vi "Untitled4.vi"() -> ()   [LabVIEW 2020]
uses:
  HAL/Source/Config from JSON/Config from JSON.lvclass
  HAL/HAL-Devices/source/Configure Strategies/PCAN-USB Strategies/PCAN-USB Read-Write Raw CAN Frame Strategy/PCAN Read-Write Raw CAN Frame Strategy.lvclass
  HAL/Source/Communicator/Communicator.lvclass
  CANopen Response/CANopen Response Message.lvclass
  CANopen Master/CANopen Master.lvclass
  CANopen Message/CANopen Message.lvclass
  <vilib>/ProgressBar/Progress Bar Dialog.lvclass
  EDS-File-Viewer/source/Electronic Datasheet/Electronic Datasheet.lvclass
panel:
  out "Success":bool[](array[boolean])
  out "Objects List":string[](array[string])
  out "Values":variant[](array[variant])
  in  "Actual Values Button":bool
  out "Uploaded":variant
  out "MSG Log":string
  in  "Discover Button":bool
  out "Success? DL":bool
  in  "Value":u16
  in  "Multiplexer DL":cluster{"Index":u16, "Sub-Index":u8} {"Index" format="%.0x"}
  in  "Download Button":bool
  in  "Node-ID DL":u8
  out "Available Nodes":map{u8, u8}(c390)
  out "Success? UL":bool
  out "Data UL":u8[](array[numeric]) format="%.0x"
  in  "Node-ID UPL":u8
  in  "Multiplexer":cluster{"Index":u16, "Sub-Index":u8} {"Index" format="%.0x"}
  in  "Upload Button":bool
  out "Emergency?":bool[](array[boolean])
  out "Nodes":u8[](array[numeric])
  in  "stop":bool
  out "Timed Outs?":bool[](array[boolean])
  out "Node-IDs":u8[](array[numeric])
  out "error out":errorcluster
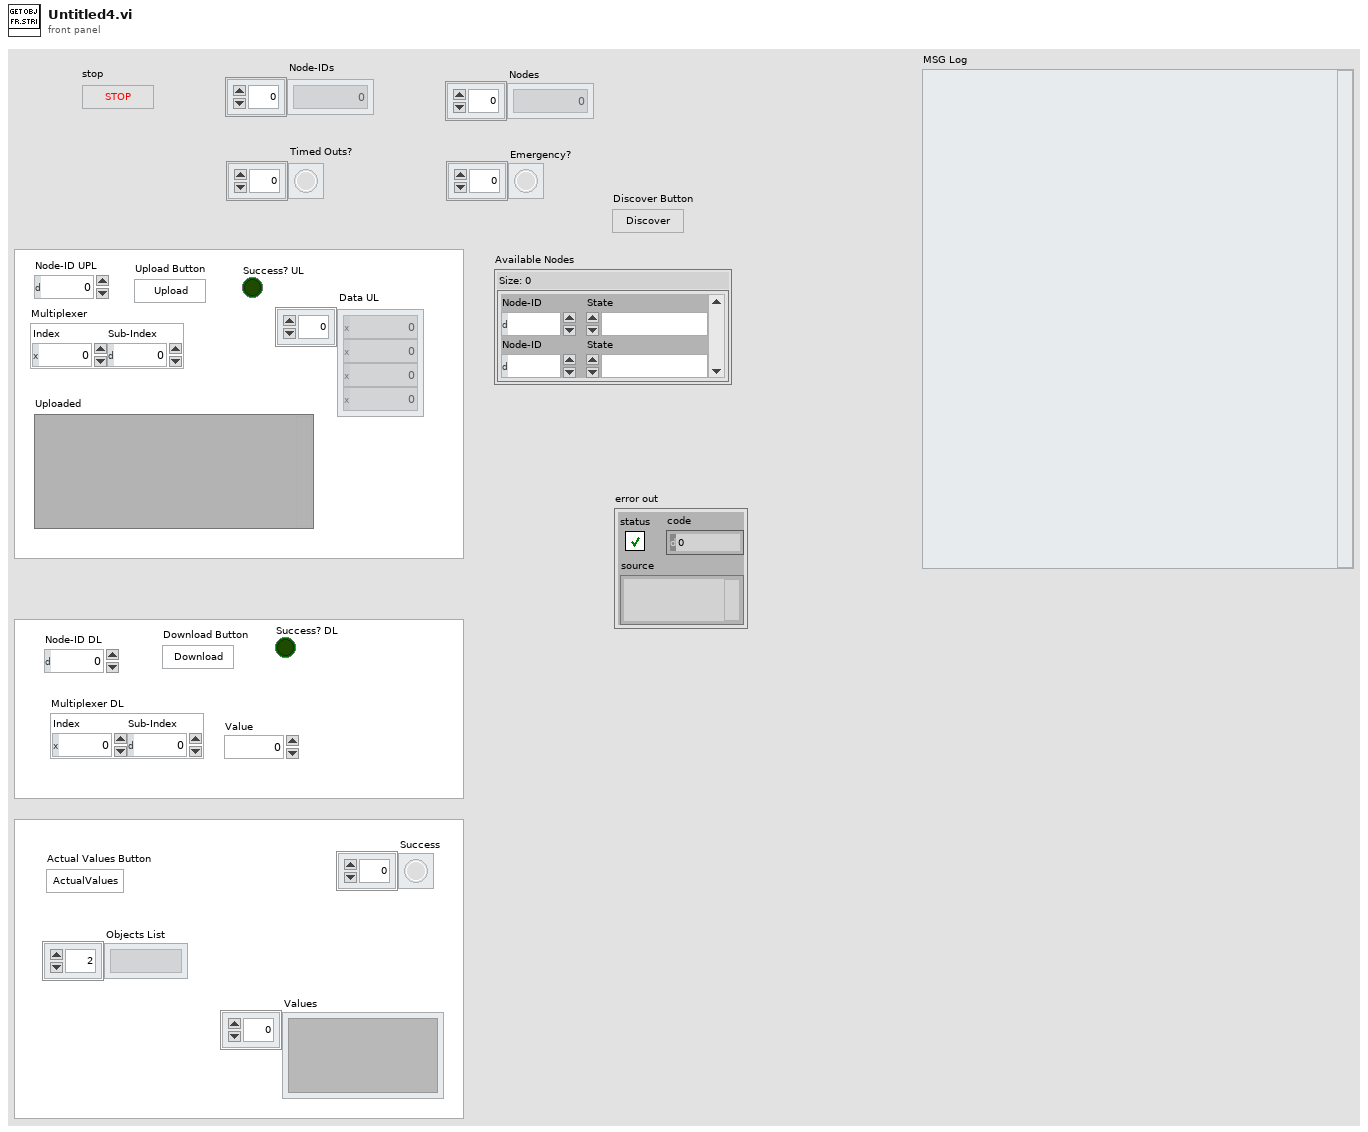
[diagram p1: front panel]
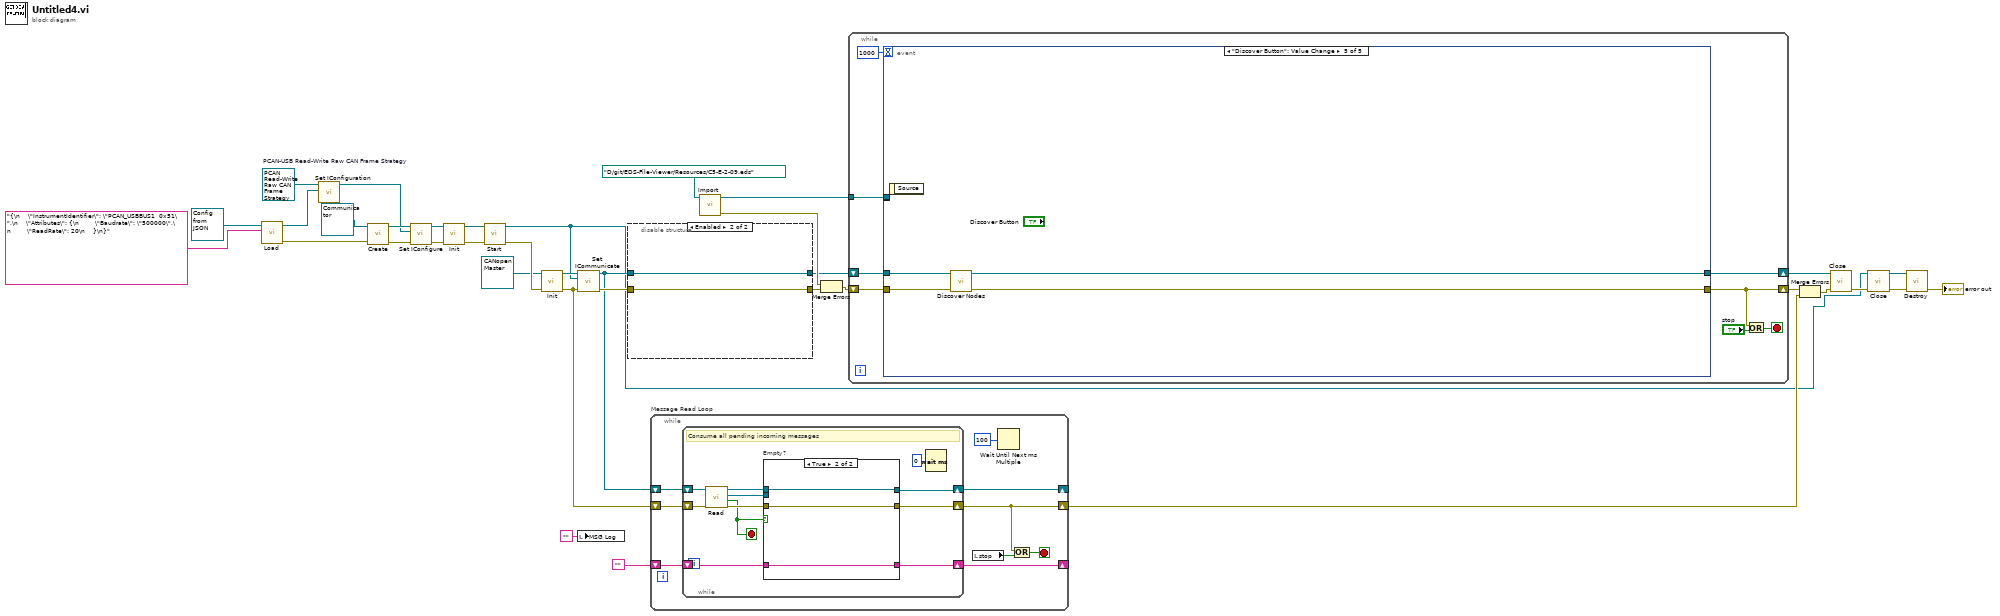
[diagram p0: block diagram]
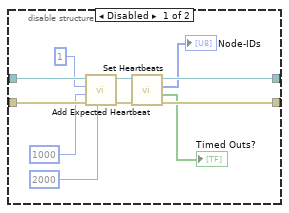
[diagram p2: hidden frame]
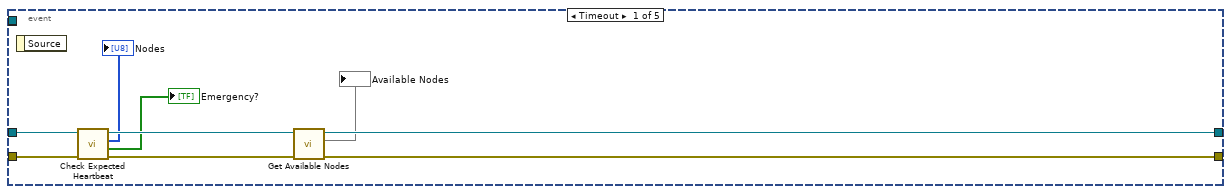
[diagram p3: hidden frame]
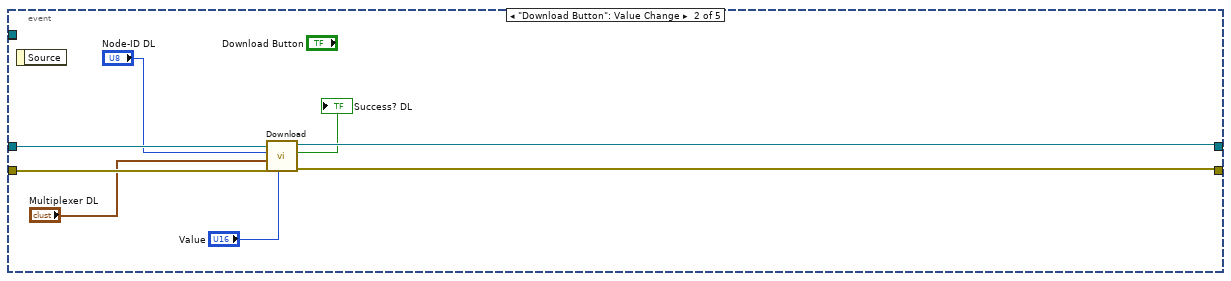
[diagram p4: hidden frame]
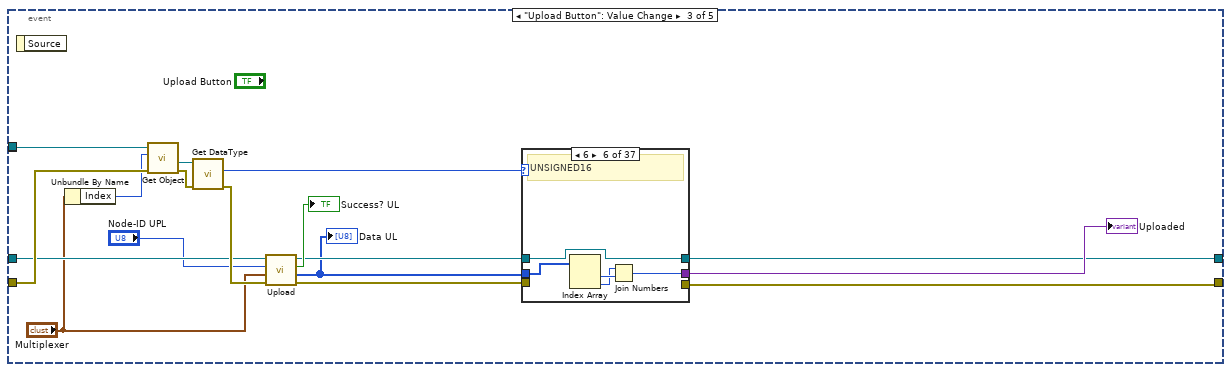
[diagram p5: hidden frame]
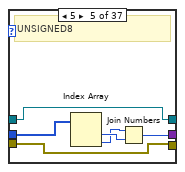
[diagram p10: hidden frame]
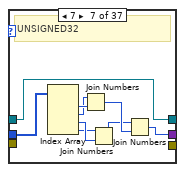
[diagram p11: hidden frame]
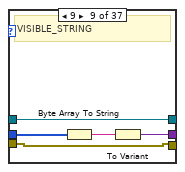
[diagram p13: hidden frame]
diagram:
  w8 = refnum<class "PCAN Read-Write Raw CAN Frame Strategy.lvclass"> refnum  # PCAN-USB Read-Write Raw CAN Frame Strategy
  n1 = call-dynamic "Load.vi"("Source"="{\n    \"InstrumentIdentifier\": \"PCAN_USBBUS1  0x51\",\n    \"Attributes\": {\n        \"Baudrate\": \"500000\",\n        \"ReadRate\": 20\n    }\n}" ("<JSON>CFG"), "Config From JSON in"=refnum<class "Config from JSON.lvclass"> refnum ("Config from JSON.lvclass")) -> ("error out"=w22:errorcluster, "Config From JSON out"=w5:refnum<class "Config from JSON.lvclass">)  [unwired: 8 in]
  n2 = call-dynamic "Set IConfiguration.vi"("IConfiguration"=w5, "PCAN-USB Read-Write Raw CAN Frame Strategy in"=w8) -> ("PCAN-USB Read-Write Raw CAN Frame Strategy out"=w4:refnum<class "PCAN Read-Write Raw CAN Frame Strategy.lvclass">)  [unwired: 9 in]
  n3 = call-dynamic "Create.vi"("Error In"=w22, "reference in"=refnum<class "Communicator.lvclass"> refnum ("Communicator")) -> ("Error Out"=w26:errorcluster, "reference out"=w9:refnum<class "Communicator.lvclass">)  [unwired: 8 in]
  n4 = call-dynamic "Set IConfigure.vi"("Error In"=w26, "IConfigure"=w4, "Communicator in"=w9) -> ("Error Out"=w25:errorcluster, "Communicator out"=w19:refnum<class "Communicator.lvclass">)  [unwired: 7 in]
  n5 = call-dynamic "Init.vi"("Error In"=w25, "Communicator in"=w19) -> ("Error Out"=w23:errorcluster, "Communicator out"=w2:refnum<class "Communicator.lvclass">)  [unwired: 8 in]
  n6 = call-dynamic "Start.vi"("Error In"=w23, "Communicator in"=w2) -> ("Error Out"=w21:errorcluster, "Communicator out"=w1:refnum<class "Communicator.lvclass">)  [unwired: 8 in]
  n7 = call "Init.vi"("error in"=w21, "CANopen Master in"=refnum<class "CANopen Master.lvclass"> refnum ("CANopen Master.lvlib:CANopen Master")) -> ("error out"=w33:errorcluster, "CANopen Master out"=w18:refnum<class "CANopen Master.lvclass">)  [unwired: 8 in]
  n8 = call "Set ICommunicate.vi"("ICommunicate"=w1, "CANopen Master in"=w18) -> ("CANopen Master out"=w17:refnum<class "CANopen Master.lvclass">)  [unwired: 8 in, 1 out]
  n9 = local write "MSG Log"("") -> ()
  n10 = disable-structure shown="Enabled" {
    disable-tunnel: w33 -> [w46 w48]
    disable-tunnel: w17 -> [w43 w47]
    disable-tunnel: [w42 w47] -> w16
    disable-tunnel: [w45 w48] -> w30
    frame Disabled {
      n11 = call "Add Expected Heartbeat.vi"("Timeout"=u16 2000, "error in"=w46, "Period"=u16 1000, "Node-ID"=u8 1, "CANopen Master in"=w43) -> ("error out"=w44:errorcluster, "CANopen Master out"=w38:refnum<class "CANopen Master.lvclass">)  [unwired: 5 in]
      n12 = call "Set Heartbeats.vi"("error in"=w44, "CANopen Master in"=w38) -> ("error out"=w45:errorcluster, "Timed Outs?"=→"Timed Outs?":bool[], "Node-IDs"=→"Node-IDs":u8[], "CANopen Master out"=w42:refnum<class "CANopen Master.lvclass">)  [unwired: 6 in]
    }
    frame Enabled {
    }
  }
  n13 = while "Message Read Loop" {
    shift-right: [w56] -> w31
    shift-left: w33 -> [w57]
    shift-right: [w53] -> _
    shift-left: w17 -> [w55]
    shift-right: [w49] -> _
    shift-left: "" -> [w50]
    stop <- w54 stop-if-true
    n14 = while {
      shift-right: [w67] -> w56
      shift-left: w57 -> [w68]
      shift-right: [w61] -> w53
      shift-left: w55 -> [w65]
      shift-right: [w58] -> w49
      shift-left: w50 -> [w59]
      stop <- w60 stop-if-true
      # "Consume all pending incoming messages"
      n15 = call "Read.vi"("error in"=w68, "CANopen Master in"=w65) -> ("error out"=w66:errorcluster, "Empty?"=w60:bool, "CANopen Message out"=w64:refnum<class "CANopen Response Message.lvclass">, "CANopen Master out"=w62:refnum<class "CANopen Master.lvclass">)  [unwired: 6 in]
      n16 = case "Empty?" shown="True" w60 {
        tunnel: w64 -> [w71 _]
        tunnel: [w76 w80] -> w67
        tunnel: w66 -> [w77 w80]
        tunnel: w62 -> [w75 w79]
        tunnel: [w74 w79] -> w61
        tunnel: w59 -> [w72 w78]
        tunnel: [w69 w78] -> w58
        frame False {
          n17 = call "Print.vi"("CANopen Message in"=w71) -> ("Message"=w70:string)  [unwired: 9 in, 1 out]
          n18 = call "React.vi"("error in"=w77, "CANopen Message"=w71, "CANopen Master in"=w75) -> ("error out"=w76:errorcluster, "CANopen Master out"=w74:refnum<class "CANopen Master.lvclass">)  [unwired: 7 in]
          n19 = Concatenate Strings(w70, "\r", w72) -> (w69:string)
          "MSG Log" <- w69
        }
        frame True {
        }
      }
      n20 = Wait (ms)(milliseconds to wait=u32 0) -> ()  [unwired: 1 out]
    }
    n21 = local read "stop"() -> (w51:bool)
    n22 = Wait Until Next ms Multiple(millisecond multiple=100) -> ()  [unwired: 1 out]
    n23 = Or(x=w56, y=w51) -> (x .or. y?=w54:bool)
  }
  n24 = call "Import.vi"("EDS File Path"=path "D:/git/EDS-File-Viewer/Resources/C5-E-2-09.eds") -> ("error out"=w27:errorcluster, "Electronic Datasheet"=w11:refnum<class "Electronic Datasheet.lvclass">)  [unwired: 9 in]
  n25 = Merge Errors(w27, w30) -> (w28:errorcluster)
  n26 = while {
    shift-right: [w84] -> w15
    shift-left: w16 -> [w85]
    shift-right: [w87] -> w29
    shift-left: w28 -> [w88]
    tunnel: w11 -> [w81]
    stop <- w83 stop-if-true
    n27 = event shown="[4] \"Discover Button\": Value Change" {
      selector: _ -> [_ _ _ _ _]
      dyn-events: _ -> [_ _ _ _ _]
      timeout: 1000 -> [_ _ _ _ _]
      tunnel: w85 -> [w94 w102 w116 w156 w261]
      tunnel: w88 -> [w96 w104 w118 w159 w263]
      tunnel: [w95 w103 w120 w157 w262] -> w87
      tunnel: [w90 w101 w108 _ w260] -> w84
      tunnel: w81 -> [_ _ w114 w148 _]
      tunnel: [_ _ w114 _ _] -> _
      event Timeout {
        n28 = event-data() -> ()  [unwired: 1 in, 1 out]
        n29 = call "Check Expected Heartbeat.vi"("error in"=w96, "CANopen Master in"=w94) -> ("error out"=w95:errorcluster, "Emergency?"=→"Emergency?":bool[], "Nodes"=→"Nodes":u8[], "CANopen Master out"=w93:refnum<class "CANopen Master.lvclass">)  [unwired: 6 in]
        n30 = call "Get Available Nodes.vi"("CANopen Master in"=w93) -> ("Nodes"=→"Available Nodes":map{u8, u8}, "CANopen Master out"=w90:refnum<class "CANopen Master.lvclass">)  [unwired: 8 in, 1 out]
      }
      event "Download Button": Value Change {
        n31 = event-data() -> ()  [unwired: 1 in, 1 out]
        n32 = call "Download.vi"("Value"="Value", "error in"=w104, "Multiplexer"="Multiplexer DL", "Node-ID"="Node-ID DL", "CANopen Master in"=w102) -> ("error out"=w103:errorcluster, "Success?"=→"Success? DL":bool, "CANopen Master out"=w101:refnum<class "CANopen Master.lvclass">)  [unwired: 4 in]
      }
      event "Upload Button": Value Change {
        n33 = event-data() -> ()  [unwired: 1 in, 1 out]
        n34 = Unbundle By Name("Multiplexer") -> ("Index"=w107:u16)
        n35 = call "Get Object.vi"("error in"=w118, "Index"=w107, "reference in"=w114) -> ("error out"=w119:errorcluster, "OD Entry"=w106:refnum<class "OD Entry.lvclass">)  [unwired: 5 in, 2 out]
        n36 = call "Get DataType.vi"("Error In"=w119, "reference in"=w106) -> ("Error Out"=w117:errorcluster, "DataType"=w105:u16)  [unwired: 7 in, 1 out]
        n37 = call "Upload.vi"("error in"=w117, "Multiplexer"="Multiplexer", "Node-ID"="Node-ID UPL", "CANopen Master in"=w116) -> ("error out"=w121:errorcluster, "Value"=w110:u8[], "Success?"=→"Success? UL":bool, "CANopen Master out"=w111:refnum<class "CANopen Master.lvclass">)  [unwired: 4 in]
        "Data UL" <- w110
        n38 = case shown="6" w105 {
          tunnel: w111 -> [_ _ _ _ w125 w128 w133 _ w143 _ _ _ _ _ _ _ _ _ _ _ _ _ _ _ _ _ _ _ _ _ _ _ _ _ _ _ _]
          tunnel: w121 -> [_ _ _ _ w127 _ _ _ w146 _ _ _ _ _ _ _ _ _ _ _ _ _ _ _ _ _ _ _ _ _ _ _ _ _ _ _ _]
          tunnel: w110 -> [_ _ _ _ w126 w132 w141 _ w145 _ _ _ _ _ _ _ _ _ _ _ _ _ _ _ _ _ _ _ _ _ _ _ _ _ _ _ _]
          tunnel: [_ _ _ _ w122 w129 w134 _ w142 _ _ _ _ _ _ _ _ _ _ _ _ _ _ _ _ _ _ _ _ _ _ _ _ _ _ _ _] -> w109
          tunnel: [_ _ _ _ w127 _ _ _ w146 _ _ _ _ _ _ _ _ _ _ _ _ _ _ _ _ _ _ _ _ _ _ _ _ _ _ _ _] -> w120
          tunnel: [_ _ _ _ w125 w128 w133 _ w143 _ _ _ _ _ _ _ _ _ _ _ _ _ _ _ _ _ _ _ _ _ _ _ _ _ _ _ _] -> w108
          frame 1 {
            # "BOOLEAN"
          }
          frame 2 {
            # "INTEGER8"
          }
          frame 3 {
            # "INTEGER16"
          }
          frame 4 {
            # "INTEGER32"
          }
          frame 5 {
            # "UNSIGNED8"
            n39 = Index Array(array=w126) -> (element #1=w124:u8, element #2=w123:u8)  [unwired: 2 in]
            n40 = Join Numbers(hi=w123, lo=w124) -> ((hi.lo)=w122:u16)
          }
          frame 6 {
            # "UNSIGNED16"
            n41 = Index Array(array=w132) -> (element #1=w131:u8, element #2=w130:u8)  [unwired: 2 in]
            n42 = Join Numbers(hi=w130, lo=w131) -> ((hi.lo)=w129:u16)
          }
          frame 7 {
            # "UNSIGNED32"
            n43 = Index Array(array=w141) -> (element #1=w140:u8, element #2=w139:u8, element #3=w138:u8, element #4=w137:u8)  [unwired: 4 in]
            n44 = Join Numbers(hi=w139, lo=w140) -> ((hi.lo)=w136:u16)
            n45 = Join Numbers(hi=w137, lo=w138) -> ((hi.lo)=w135:u16)
            n46 = Join Numbers(hi=w135, lo=w136) -> ((hi.lo)=w134:u32)
          }
          frame 8 {
            # "REAL32"
          }
          frame 9 {
            # "VISIBLE_STRING"
            n47 = Byte Array To String(unsigned byte array=w145) -> (string=w144:string)
            n48 = To Variant(anything=w144) -> (Variant=w142:variant)
          }
          frame 10 {
            # "OCTET_STRING"
          }
          frame 11 {
            # "UNICODE_STRING"
          }
          frame 12 {
            # "TIME_OF_DAY"
          }
          frame 13 {
            # "TIME_DIFFERENCE"
          }
          frame 14 {
            # "RESERVED1"
          }
          frame 15 {
            # "DOMAIN"
          }
          frame 16 {
            # "INTEGER24"
          }
          frame 17 {
            # "REAL64"
          }
          frame 18 {
            # "INTEGER40"
          }
          frame 19 {
            # "INTEGER48"
          }
          frame 20 {
            # "INTEGER56"
          }
          frame 21 {
            # "INTEGER64"
          }
          frame 22 {
            # "UNSIGNED24"
          }
          frame 23 {
            # "RESERVED2"
          }
          frame 24 {
            # "UNSIGNED40"
          }
          frame 25 {
            # "UNSIGNED48"
          }
          frame 26 {
            # "UNSIGNED56"
          }
          frame 27 {
            # "UNSIGNED64"
          }
          frame 28 {
            # "RESERVED3"
          }
          frame 29 {
            # "RESERVED4"
          }
          frame 30 {
            # "RESERVED5"
          }
          frame 31 {
            # "RESERVED6"
          }
          frame 32 {
            # "PDO_COMMUNICATION_PARAMETER"
          }
          frame 33 {
            # "PDO_MAPPING"
          }
          frame 34 {
            # "SDO_PARAMETER"
          }
          frame 35 {
            # "IDENTITY"
          }
          frame 36 {
            # "RESERVED7"
          }
          frame Default {
            # "INVALID"
          }
        }
        "Uploaded" <- w109
      }
      event "Actual Values Button": Value Change {
        n49 = event-data() -> ()  [unwired: 1 in, 1 out]
        n50 = call "Get Communication Specific Objects.vi"("error in"=w159, "Electronic Datasheet"=w148) -> ("error out"=w158:errorcluster, "Entries"=w147:refnum<class "OD Entry.lvclass">[])  [unwired: 7 in, 1 out]
        n51 = local read "Node-ID UPL"() -> (w150:u8)
        n52 = Array Size(array=w147) -> (size(s)=w153:i32)
        n53 = call <vilib>:"Launch Progress Bar.vi"("Main Title (\"Working...\")"="Uploading Actual Values" ("Main Title (\"Working...\")"), "Total Count"=w153) -> ("Progress Bar Dialog"=w155:refnum<class "Progress Bar Dialog.lvclass">)  [unwired: 8 in, 1 out]
        n54 = for {
          shift-right: [w172] -> w154
          shift-left: w155 -> [w173]
          tunnel: [w174] -> w151 mode=concatenating
          shift-right: [w171] -> _
          shift-left: w156 -> [w175]
          tunnel: w150 -> [w170]
          shift-right: [w178] -> w157
          shift-left: w158 -> [w177]
          tunnel: [w165] -> w149 mode=concatenating
          tunnel: w147 -> [w161] mode=indexing
          n55 = call "Get Index.vi"("Error In"=w177, "reference in"=w161) -> ("Error Out"=w176:errorcluster, "Index"=w164:u16, "reference out"=w162:refnum<class "OD Entry.lvclass">)  [unwired: 7 in]
          n56 = Format Into String(format string="%x", w164) -> (resulting string=w160:string)  [unwired: 2 in, 1 out]
          n57 = call "Get All Sub-Entries.vi"("Error In"=w176, "reference in"=w162) -> ("Error Out"=w179:errorcluster, "Indices"=w168:u8[], "Sub-Entries"=w167:refnum<class "OD Sub-Entry.lvclass">[], "reference out"=w166:refnum<class "OD Entry.lvclass">)  [unwired: 6 in]
          n58 = call <vilib>:"Increment Progress Bar.vi"("Step Name (\"\")"=w160, "Progress Bar Dialog in"=w173) -> ("Progress Bar Dialog out"=w172:refnum<class "Progress Bar Dialog.lvclass">)  [unwired: 7 in, 2 out]
          n59 = Array Size(array=w167) -> (size(s)=w169:i32)
          n60 = case "Index has Sub-Entries?" shown="Default" w169 {
            tunnel: w175 -> [w192 w222]
            tunnel: [w187 w219] -> w174
            tunnel: w179 -> [w194 w224]
            tunnel: w168 -> [_ w217]
            tunnel: [w186 w221] -> w171
            tunnel: w170 -> [w188 w220]
            tunnel: [w195 w223] -> w178
            tunnel: w167 -> [_ w218]
            tunnel: w166 -> [w183 _]
            tunnel: [w181 w216] -> w165
            tunnel: w160 -> [w180 w215]
            frame 0 {
              n61 = Bundle(w180, "") -> (w184:cluster{string, string})  [unwired: 1 in]
              n62 = call "Upload from String.vi"("error in"=w194, "Multiplexer"=w184, "Node-ID"=w188, "CANopen Master in"=w192) -> ("error out"=w193:errorcluster, "Value"=w191:u8[], "Success?"=w182:bool, "CANopen Master out"=w186:refnum<class "CANopen Master.lvclass">)  [unwired: 4 in]
              n63 = call "Get DataType.vi"("Error In"=w193, "reference in"=w183) -> ("Error Out"=w195:errorcluster, "DataType"=w189:u16)  [unwired: 7 in, 1 out]
              n64 = case shown="5" w189 {
                tunnel: w191 -> [_ _ _ _ w199 w203 w211 _ w214 _ _ _ _ _ _ _ _ _ _ _ _ _ _ _ _ _ _ _ _ _ _ _ _ _ _ _ _]
                tunnel: [_ _ _ _ w196 w200 w204 _ w212 _ _ _ _ _ _ _ _ _ _ _ _ _ _ _ _ _ _ _ _ _ _ _ _ _ _ _ _] -> w190
                frame 1 {
                  # "BOOLEAN"
                }
                frame 2 {
                  # "INTEGER8"
                }
                frame 3 {
                  # "INTEGER16"
                }
                frame 4 {
                  # "INTEGER32"
                }
                frame 5 {
                  # "UNSIGNED8"
                  n65 = Index Array(array=w199) -> (element #1=w198:u8, element #2=w197:u8)  [unwired: 2 in]
                  n66 = Join Numbers(hi=w197, lo=w198) -> ((hi.lo)=w196:u16)
                }
                frame 6 {
                  # "UNSIGNED16"
                  n67 = Index Array(array=w203) -> (element #1=w202:u8, element #2=w201:u8)  [unwired: 2 in]
                  n68 = Join Numbers(hi=w201, lo=w202) -> ((hi.lo)=w200:u16)
                }
                frame 7 {
                  # "UNSIGNED32"
                  n69 = Index Array(array=w211) -> (element #1=w210:u8, element #2=w209:u8, element #3=w208:u8, element #4=w207:u8)  [unwired: 4 in]
                  n70 = Join Numbers(hi=w209, lo=w210) -> ((hi.lo)=w206:u16)
                  n71 = Join Numbers(hi=w207, lo=w208) -> ((hi.lo)=w205:u16)
                  n72 = Join Numbers(hi=w205, lo=w206) -> ((hi.lo)=w204:u32)
                }
                frame 8 {
                  # "REAL32"
                }
                frame 9 {
                  # "VISIBLE_STRING"
                  n73 = Byte Array To String(unsigned byte array=w214) -> (string=w213:string)
                  n74 = To Variant(anything=w213) -> (Variant=w212:variant)
                }
                frame 10 {
                  # "OCTET_STRING"
                }
                frame 11 {
                  # "UNICODE_STRING"
                }
                frame 12 {
                  # "TIME_OF_DAY"
                }
                frame 13 {
                  # "TIME_DIFFERENCE"
                }
                frame 14 {
                  # "RESERVED1"
                }
                frame 15 {
                  # "DOMAIN"
                }
                frame 16 {
                  # "INTEGER24"
                }
                frame 17 {
                  # "REAL64"
                }
                frame 18 {
                  # "INTEGER40"
                }
                frame 19 {
                  # "INTEGER48"
                }
                frame 20 {
                  # "INTEGER56"
                }
                frame 21 {
                  # "INTEGER64"
                }
                frame 22 {
                  # "UNSIGNED24"
                }
                frame 23 {
                  # "RESERVED2"
                }
                frame 24 {
                  # "UNSIGNED40"
                }
                frame 25 {
                  # "UNSIGNED48"
                }
                frame 26 {
                  # "UNSIGNED56"
                }
                frame 27 {
                  # "UNSIGNED64"
                }
                frame 28 {
                  # "RESERVED3"
                }
                frame 29 {
                  # "RESERVED4"
                }
                frame 30 {
                  # "RESERVED5"
                }
                frame 31 {
                  # "RESERVED6"
                }
                frame 32 {
                  # "PDO_COMMUNICATION_PARAMETER"
                }
                frame 33 {
                  # "PDO_MAPPING"
                }
                frame 34 {
                  # "SDO_PARAMETER"
                }
                frame 35 {
                  # "IDENTITY"
                }
                frame 36 {
                  # "RESERVED7"
                }
                frame Default {
                  # "INVALID"
                }
              }
              n75 = Build Array(w182) -> (w181:bool[])
              n76 = Build Array(w190) -> (w187:variant[])
            }
            frame Default {
              n77 = for {
                shift-right: [w236] -> w221
                shift-left: w222 -> [w237]
                tunnel: w220 -> [w235]
                tunnel: w215 -> [w234]
                shift-right: [w238] -> w223
                shift-left: w224 -> [w240]
                tunnel: w218 -> [w231] mode=indexing
                tunnel: [w229] -> w219 mode=indexing
                tunnel: w217 -> [w226] mode=indexing
                tunnel: [w225] -> w216 mode=indexing
                n78 = Format Into String(format string="%d", w226) -> (resulting string=w227:string)  [unwired: 2 in, 1 out]
                n79 = Bundle(w234, w227) -> (w233:cluster{string, string})  [unwired: 1 in]
                n80 = call "Upload from String.vi"("error in"=w240, "Multiplexer"=w233, "Node-ID"=w235, "CANopen Master in"=w237) -> ("error out"=w239:errorcluster, "Value"=w230:u8[], "Success?"=w225:bool, "CANopen Master out"=w236:refnum<class "CANopen Master.lvclass">)  [unwired: 4 in]
                n81 = call "Get DataType.vi"("Error In"=w239, "reference in"=w231) -> ("Error Out"=w238:errorcluster, "DataType"=w232:u16)  [unwired: 7 in, 1 out]
                n82 = case shown="7" w232 {
                  tunnel: w230 -> [_ _ _ _ w244 w248 w256 _ w259 _ _ _ _ _ _ _ _ _ _ _ _ _ _ _ _ _ _ _ _ _ _ _ _ _ _ _ _]
                  tunnel: [_ _ _ _ w241 w245 w249 _ w257 _ _ _ _ _ _ _ _ _ _ _ _ _ _ _ _ _ _ _ _ _ _ _ _ _ _ _ _] -> w229
                  frame 1 {
                    # "BOOLEAN"
                  }
                  frame 2 {
                    # "INTEGER8"
                  }
                  frame 3 {
                    # "INTEGER16"
                  }
                  frame 4 {
                    # "INTEGER32"
                  }
                  frame 5 {
                    # "UNSIGNED8"
                    n83 = Index Array(array=w244) -> (element #1=w243:u8, element #2=w242:u8)  [unwired: 2 in]
                    n84 = Join Numbers(hi=w242, lo=w243) -> ((hi.lo)=w241:u16)
                  }
                  frame 6 {
                    # "UNSIGNED16"
                    n85 = Index Array(array=w248) -> (element #1=w247:u8, element #2=w246:u8)  [unwired: 2 in]
                    n86 = Join Numbers(hi=w246, lo=w247) -> ((hi.lo)=w245:u16)
                  }
                  frame 7 {
                    # "UNSIGNED32"
                    n87 = Index Array(array=w256) -> (element #1=w255:u8, element #2=w254:u8, element #3=w253:u8, element #4=w252:u8)  [unwired: 4 in]
                    n88 = Join Numbers(hi=w254, lo=w255) -> ((hi.lo)=w251:u16)
                    n89 = Join Numbers(hi=w252, lo=w253) -> ((hi.lo)=w250:u16)
                    n90 = Join Numbers(hi=w250, lo=w251) -> ((hi.lo)=w249:u32)
                  }
                  frame 8 {
                    # "REAL32"
                  }
                  frame 9 {
                    # "VISIBLE_STRING"
                    n91 = Byte Array To String(unsigned byte array=w259) -> (string=w258:string)
                    n92 = To Variant(anything=w258) -> (Variant=w257:variant)
                  }
                  frame 10 {
                    # "OCTET_STRING"
                  }
                  frame 11 {
                    # "UNICODE_STRING"
                  }
                  frame 12 {
                    # "TIME_OF_DAY"
                  }
                  frame 13 {
                    # "TIME_DIFFERENCE"
                  }
                  frame 14 {
                    # "RESERVED1"
                  }
                  frame 15 {
                    # "DOMAIN"
                  }
                  frame 16 {
                    # "INTEGER24"
                  }
                  frame 17 {
                    # "REAL64"
                  }
                  frame 18 {
                    # "INTEGER40"
                  }
                  frame 19 {
                    # "INTEGER48"
                  }
                  frame 20 {
                    # "INTEGER56"
                  }
                  frame 21 {
                    # "INTEGER64"
                  }
                  frame 22 {
                    # "UNSIGNED24"
                  }
                  frame 23 {
                    # "RESERVED2"
                  }
                  frame 24 {
                    # "UNSIGNED40"
                  }
                  frame 25 {
                    # "UNSIGNED48"
                  }
                  frame 26 {
                    # "UNSIGNED56"
                  }
                  frame 27 {
                    # "UNSIGNED64"
                  }
                  frame 28 {
                    # "RESERVED3"
                  }
                  frame 29 {
                    # "RESERVED4"
                  }
                  frame 30 {
                    # "RESERVED5"
                  }
                  frame 31 {
                    # "RESERVED6"
                  }
                  frame 32 {
                    # "PDO_COMMUNICATION_PARAMETER"
                  }
                  frame 33 {
                    # "PDO_MAPPING"
                  }
                  frame 34 {
                    # "SDO_PARAMETER"
                  }
                  frame 35 {
                    # "IDENTITY"
                  }
                  frame 36 {
                    # "RESERVED7"
                  }
                  frame Default {
                    # "INVALID"
                  }
                }
              }
            }
          }
        }
        "Values" <- w151
        "Success" <- w149
        n93 = call <vilib>:"Close Progress Bar.vi"("Progress Bar Dialog"=w154) -> ()  [unwired: 10 in, 1 out]
      }
      event "Discover Button": Value Change {
        n94 = event-data() -> ()  [unwired: 1 in, 1 out]
        n95 = call "Discover Nodes.vi"("error in"=w263, "CANopen Master in"=w261) -> ("error out"=w262:errorcluster, "CANopen Master out"=w260:refnum<class "CANopen Master.lvclass">)  [unwired: 8 in]
      }
    }
    n96 = Or(x=w87, y="stop") -> (x .or. y?=w83:bool)
  }
  n97 = Merge Errors(w29, w31) -> (w32:errorcluster)
  n98 = call "Close.vi"("error in"=w32, "CANopen Master in"=w15) -> ("error out"=w35:errorcluster)  [unwired: 8 in, 1 out]
  n99 = call-dynamic "Close.vi"("Error In"=w35, "Communicator in"=w1) -> ("Error Out"=w24:errorcluster, "Communicator out"=w3:refnum<class "Communicator.lvclass">)  [unwired: 8 in]
  n100 = call-dynamic "Destroy.vi"("Error In"=w24, "Communicator in"=w3) -> ("Error Out"=→"error out":errorcluster)  [unwired: 8 in, 1 out]
